vi "CumulativeIntegral.vi"(9 "Enum":enum16{"Simple Sum", "use dx"}(ring), 10 "Y":dbl[](array[numeric]), 11 "X":dbl[](array[numeric])) -> (2 "plottableBundle":cluster{"X":dbl[], "Array":dbl[]}, 3 "Cumulative Integral":dbl[](array[numeric]))   [LabVIEW 2013]
doc: "Performs a naive rectangular integration- handy for integrating spectra"
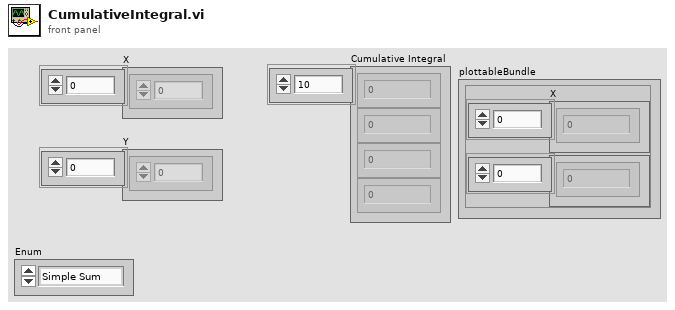
[diagram p1: front panel]
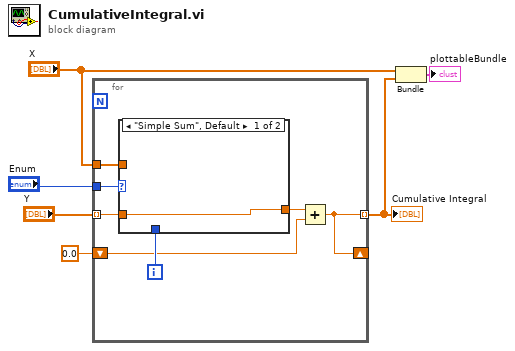
[diagram p0: block diagram]
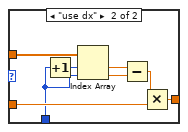
[diagram p2: hidden frame]
diagram:
  n1 = for {
    tunnel: "X" -> [w13]
    tunnel: "Y" -> [w12] mode=indexing
    tunnel: [w8] -> w4 mode=indexing
    shift-right: [w8] -> _
    shift-left: 0.0 -> [w9]
    tunnel: "Enum" -> [w7]
    i -> [w11]
    n2 = case shown="\"Simple Sum\", Default" w7 {
      tunnel: w13 -> [_ w22]
      tunnel: w12 -> [w14 w19]
      tunnel: w11 -> [_ w16]
      tunnel: [w14 w15] -> w10
      frame "Simple Sum", Default {
      }
      frame "use dx" {
        n3 = Increment(x=w16) -> (x+1=w17:i32)
        n4 = Index Array(array=w22, index #1=w17, index #2=w16) -> (element #1=w21:dbl, element #2=w20:dbl)
        n5 = Subtract(x=w21, y=w20) -> (x-y=w18:dbl)
        n6 = Multiply(x=w18, y=w19) -> (x*y=w15:dbl)
      }
    }
    n7 = Add(x=w10, y=w9) -> (x+y=w8:dbl)
  }
  "Cumulative Integral" <- w4
  n8 = Bundle("X"="X", w4) -> (→"plottableBundle":cluster{"X":dbl[], dbl[]})  [unwired: 1 in]
